vi "Write Data.vi"(8 "error in (no error)":errorcluster, 9 "Publication Time":timestamp, 10 "Value":variant, 11 "ITransport in":refnum<class "ITransport.lvclass">) -> (0 "error out":errorcluster, 3 "ITransport out":refnum<class "ITransport.lvclass">)   [LabVIEW 2017, in "IMediator.lvlib" / "ITransport.lvclass"]
doc: "<License>\nCopyright © 2017 Composed Systems, LLC | All rights reserved\nwww.composed.io\n\nAuthor: Ethan Stern <ethan.stern@composed.io>\n\nThis software is provided \"AS IS\" WITHOUT WARRANTIES, either express or implied, AND IS FOR EDUCATIONAL PURPOSES ONLY.\n</License>"
uses:
  ITransport.lvclass
  <vilib>/ErrorRing/Error Ring.xnode
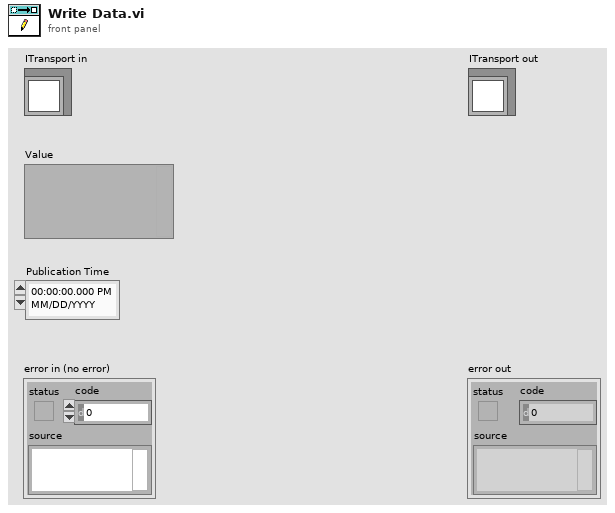
[diagram p1: front panel]
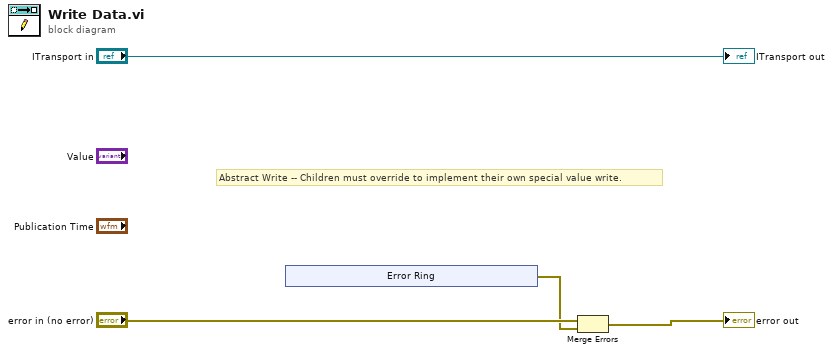
[diagram p0: block diagram]
diagram:
  # "Abstract Write -- Children must override to implement their own special value write."
  n1 = xnode "Error Ring"() -> ("error out"=w1:errorcluster)
  n2 = Merge Errors("error in (no error)", w1) -> (→"error out":errorcluster)
  "ITransport out" <- "ITransport in"
